vi "09 - Tip - Turn Off Lock Panel to Allow Asynchronicity.vi"() -> ()   [LabVIEW 2012]
panel:
  in  "Increment this to 5\nto exit the program":i32
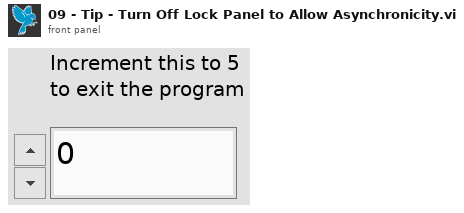
[diagram p1: front panel]
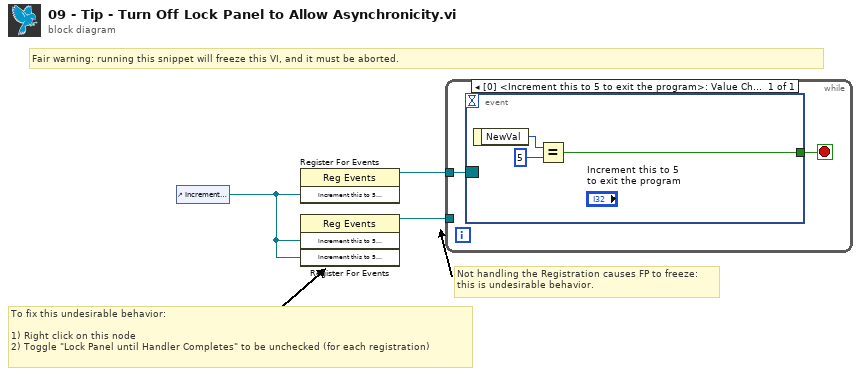
[diagram p0: block diagram]
diagram:
  # "To fix this undesirable behavior:\n\n1) Right click on this node\n2) Toggle \"Lock Panel until Handler Completes\" to be unchecked (for each registration)"
  # "Not handling the Registration causes FP to freeze:\nthis is undesirable behavior."
  # "Fair warning: running this snippet will freeze this VI, and it must be aborted."
  n1 = control-ref of="Increment this to 5\nto exit the program"() -> (w1:refnum<vi>)
  n2 = register-events(w1) -> (reference out=w3:refnum<event-registration>)  [unwired: 2 in, 1 out]
  n3 = register-events(w1, w1) -> (reference out=w2:refnum<event-registration>)  [unwired: 2 in, 1 out]
  n4 = while {
    tunnel: w3 -> [w4]
    tunnel: w2 -> [_]
    stop <- w5 stop-if-true
    n5 = event shown="[0] <Increment this to 5\nto exit the program>: Value Change" {
      selector: w4 -> [_]
      dyn-events: _ -> [_]
      timeout: _ -> [_]
      tunnel: [w6] -> w5
      event Value Change {
        n6 = event-data() -> ("NewVal"=w8:i32)  [unwired: 1 in]
        n7 = Equal?(x=w8, y=5) -> (x = y?=w6:bool)
      }
    }
  }
